vi "Send Command.vi"(7 "Data":string, 8 "error in (no error)":errorcluster, 9 "Device and Axis":string, 10 "Command":string, 11 "VISA resource name":refnum<visa-resource-name>) -> (0 "error out":errorcluster, 1 "Response Bundle Array":T1(array[cluster]), 2 "Response String Array":string[](array[string]), 3 "VISA resource name out":refnum<visa-resource-name>, 5 "Number of Replies":i32)   [LabVIEW 2011, in "Zaber A Series.lvlib"]
doc: "Sends a command to the device. For inputting the command, it combines the Device and Axis input, Command input, and Data value input to create a complete command. You could optionally send the complete command directly to the Command input. Omitting the Device and Axis will send the command to all devices/axes. See a command reference here: http://www.zaber.com/wiki/Manuals/ASCII_Protocol_Manual#Command_Reference.\n\nThe Detect Devices VI is designed to provide an easy list of valid Device and Axis inputs. \n\nAn array containing the complete strings of the responses is returned on the Response String Array output, and the details of the format of the response are described here: http://www.zaber.com/wiki/Manuals/ASCII_Protocol_Manual#Replies. This VI also parses the strings, bundles the components, and returns them as an array of bundles on the Response Bundle Array pin. Additionally a pin returns the number of responses received. \n\nThis VI requires that the Initialize VI has been called with the same serial port."
uses:
  Zaber A Series.lvlib
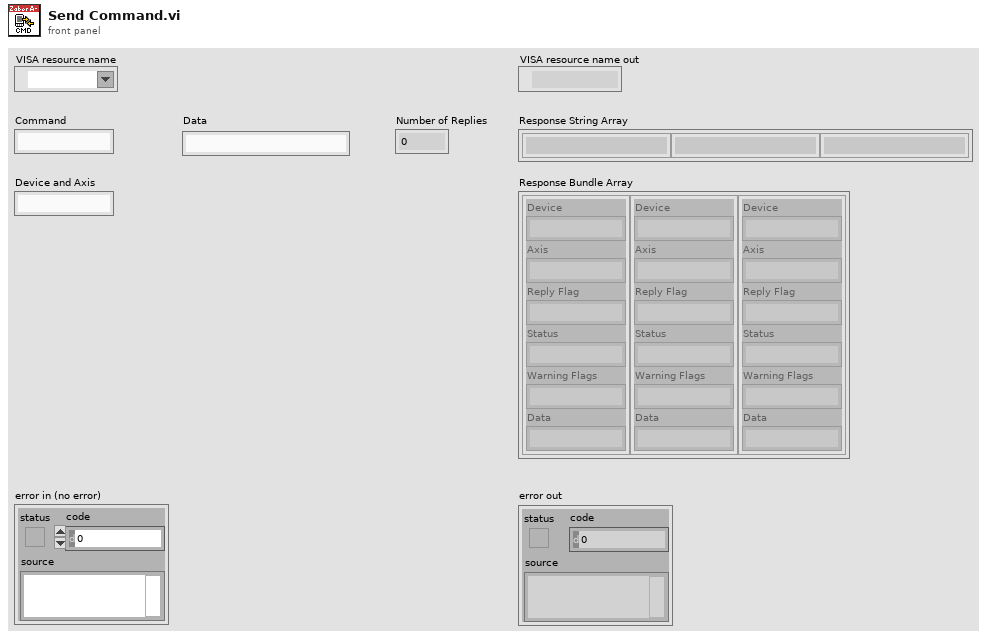
[diagram p1: front panel]
types:
  T1 = cluster{"Device":string, "Axis":string, "Reply Flag":string, "Status":string, "Warning Flags":string, "Data":string}[]
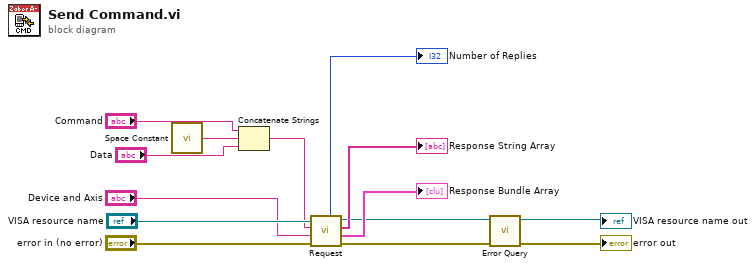
[diagram p0: block diagram]
diagram:
  n1 = call <vilib>:"Space Constant.vi"() -> ("String"=w11:string)
  n2 = Concatenate Strings("Command", w11, "Data") -> (w8:string)
  n3 = call "Request.vi"("error in (no error)"="error in (no error)", "Device and Axis"="Device and Axis", "Command String"=w8, "VISA resource name"="VISA resource name") -> ("error out"=w3:errorcluster, "Response Bundle Array"=→"Response Bundle Array":T1, "Response String Array"=→"Response String Array":string[], "VISA resource name out"=w4:refnum<visa-resource-name>, "Number of Replies"=→"Number of Replies":i32)  [unwired: 3 in]
  n4 = call "Error Query.vi"("error in (no error)"=w3, "VISA resource name"=w4) -> ("error out"=→"error out":errorcluster, "VISA resource name out"=→"VISA resource name out":refnum<visa-resource-name>)  [unwired: 6 in, 2 out]
